vi "SwissSPAD Live_Get Next Series Step.vi"(8 "error in (no error)":errorcluster, 11 "SwissSPAD Live Internal Variables in":T1={"okCFrontPanelDevices Refnum"=refnum, "Bottom Device Refnum"=refnum, "Display Image"=refnum, "# Live Images"=0, "relative s"=0.0, "# Image Sets"=0, "Message"="", "Current Image Set"=0, "# Datasets in Series"=0, "Current Dataset"=0, "Live Mode"=FALSE, "Recording Mode"=FALSE, "Record Button"=refnum, "\nLive Button"=refnum, "SwissSPAD Live Gate Image Data Q Name"="SS2 Live Gate Data Q", "Discard First Image"=FALSE, "Image Information"={"Save ROI Only"=FALSE, "Left"=0, "Top"=0, "Right"=0, "Bottom"=0, "Use Current ROI"=FALSE}, "Image Binning Options"={"Use Image Binning"=FALSE, "X Bin"=1, "Y Bin"=1}, "Bottom FPGA Serial Number"="", "Detector PCB Version"=enum."SS2 PCB1", "# Acquisitions"=1, "10 bits"=FALSE, "Top FPGA Serial Number"="", "Top Device Refnum"=refnum} {"# Acquisitions" min=1; "Image Binning Options"."Y Bin" min=1; "Image Binning Options"."X Bin" min=1}) -> (0 "Error Out":errorcluster, 1 "Message out":string, 2 "SwissSPAD Live Atomic Action":T6[](array[typedef]), 3 "SwissSPAD Live Internal Variables out":T1={"okCFrontPanelDevices Refnum"=refnum, "Bottom Device Refnum"=refnum, "Display Image"=refnum, "# Live Images"=0, "relative s"=0.0, "# Image Sets"=0, "Message"="", "Current Image Set"=0, "# Datasets in Series"=0, "Current Dataset"=0, "Live Mode"=FALSE, "Recording Mode"=FALSE, "Record Button"=refnum, "\nLive Button"=refnum, "SwissSPAD Live Gate Image Data Q Name"="SS2 Live Gate Data Q", "Discard First Image"=FALSE, "Image Information"={"Save ROI Only"=FALSE, "Left"=0, "Top"=0, "Right"=0, "Bottom"=0, "Use Current ROI"=FALSE}, "Image Binning Options"={"Use Image Binning"=FALSE, "X Bin"=1, "Y Bin"=1}, "Bottom FPGA Serial Number"="", "Detector PCB Version"=enum."SS2 PCB1", "# Acquisitions"=1, "10 bits"=FALSE, "Top FPGA Serial Number"="", "Top Device Refnum"=refnum} {"# Acquisitions" min=1; "Image Binning Options"."Y Bin" min=1; "Image Binning Options"."X Bin" min=1})   [LabVIEW 2021]
uses:
  SwissSPAD Live_Q [Element].ctl
  SwissSPAD Live_Q Event List.ctl
  SwissSPAD Live_Internal Variables.ctl
  D:/UCLA Thinkpad Google Drive/LabVIEW 2021 SP1/builds/SwissSPAD Live Distribution/Opal Kelly/C# Wrapper/v5.0.2/libFrontPanel-csharp.dll
  Opal Kelly/C# Wrapper/v5.0.2/libFrontPanel-csharp.dll
  <vilib>/vision/Image Controls.llb/IMAQ Image.ctl
  SwissSPAD Live_Image ROI Information.ctl
  Phasor/Image Binning Options.ctl
  SwissSPAD Live_SSx PCB Version.ctl
  SwissSPAD Live_Settings List.ctl
  SwissSPAD Live_File Information.ctl
  Variant/Variant to Data/Variant to Data.lvlib
  Notebook/Notebook.lvlib
  Rich Text Box/Rich Text Box.lvlib
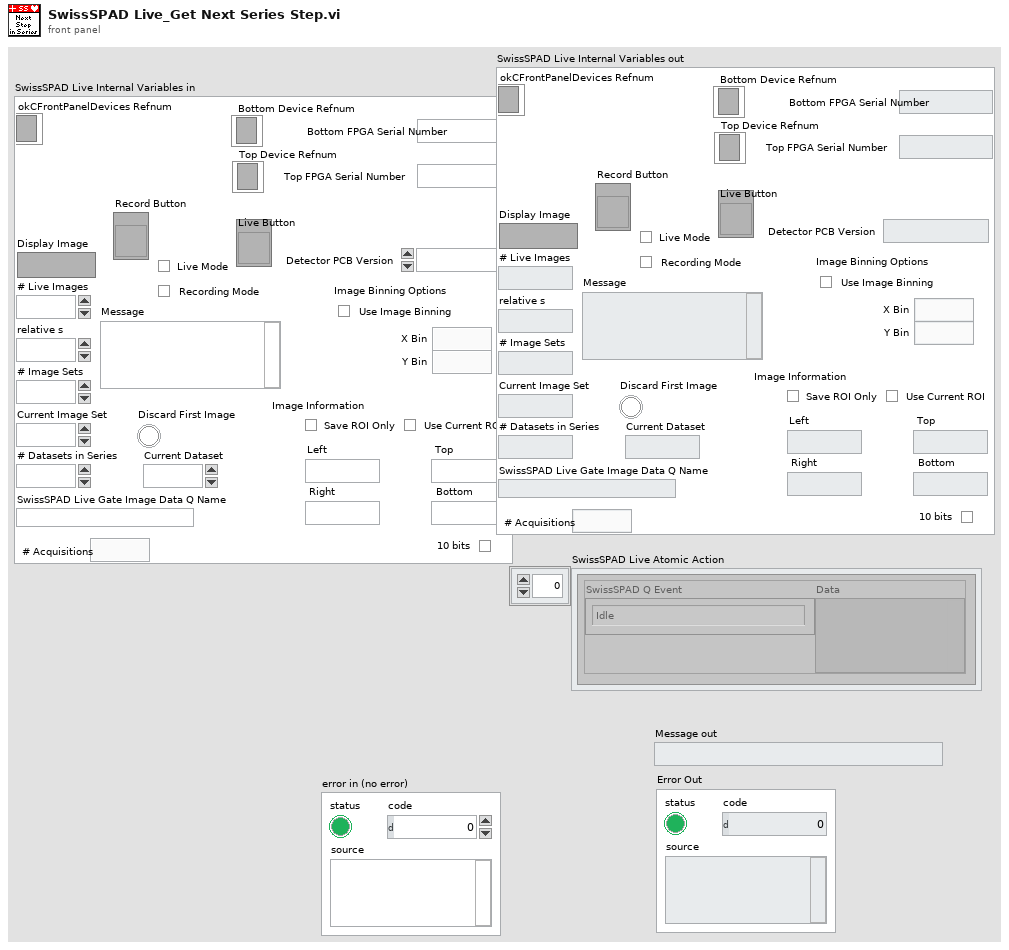
[diagram p1: front panel]
types:
  T1 = typedef "SwissSPAD Live_Internal Variables.ctl" = cluster{"okCFrontPanelDevices Refnum":refnum<k24>, "Bottom Device Refnum":refnum<k24>, "Display Image":T2, "# Live Images":i32, "relative s":dbl, "# Image Sets":i32, "Message":string, "Current Image Set":i32, "# Datasets in Series":i32, "Current Dataset":i32, "Live Mode":bool, "Recording Mode":bool, "Record Button":refnum<vi>, "\nLive Button":refnum<vi>, "SwissSPAD Live Gate Image Data Q Name":string, "Discard First Image":bool, "Image Information":T3, "Image Binning Options":T4, "Bottom FPGA Serial Number":string, "Detector PCB Version":T5, "# Acquisitions":u32, "10 bits":bool, "Top FPGA Serial Number":string, "Top Device Refnum":refnum<k24>}
  T2 = typedef "IMAQ Image.ctl" = refnum<image>
  T3 = typedef "SwissSPAD Live_Image ROI Information.ctl" = cluster{"Save ROI Only":bool, "Left":u16, "Top":u16, "Right":u16, "Bottom":u16, "Use Current ROI":bool}
  T4 = typedef "Image Binning Options.ctl" = cluster{"Use Image Binning":bool, "X Bin":i32, "Y Bin":i32}
  T5 = typedef "SwissSPAD Live_SSx PCB Version.ctl" = enum16{"unknown", "SS2 PCB1", "SS2 PCB2", "SS3 PCB1"}
  T6 = typedef "SwissSPAD Live_Q [Element].ctl" = cluster{"SwissSPAD Q Event":T7, "Data":variant}
  T7 = typedef "SwissSPAD Live_Q Event List.ctl" = enum16{"---- UI ----", "Idle", "Initialization", "Init FPGA(s)", "Init Top FPGA (deprecated)", "FPGA(s) Status", "Top FPGA Status (deprecated)", "Reset FPGA(s)", "Reset Top FPGA (deprecated)", "Refresh Display Image", "Quit", "---- DAQ ----", "Start Recording", "Start Live Acquisition", "Initialize Recording Mode", "Initialize FPGA (Live Mode)", "Get Image Set", "Get Single Image", "Update Image Display", "Stop Live Acquisition", "Stop Data Recording", "Stop Data Saving", "---- Image ----", "Copy Data to Clipboard", "Set Image Palette", "Save Displayed Image with Overlay", "Save Image Data as TIFF"}
  T8 = typedef "SwissSPAD Live_Settings List.ctl" = enum16{"FPGA:Bottom Half", "FPGA:Top Half", "FPGA:Bottom Bitfile Path", "FPGA:Top Bitfile Path", "FPGA:Bottom Bitstream Version", "FPGA:Top Bitstream Version", "FPGA:Auto Reset FPGA", "FPGA:Bottom FPGA Serial Number", "FPGA:Top FPGA Serial Number", "FPGA:Detector PCB Version", "Acquisition Parameters:Microlens", "Acquisition Parameters:SS2 DAQ Parameters", "Acquisition Parameters:Gate Configuration Array", "Acquisition Parameters:SS3 DAQ Parameters", "Acquisition Parameters:Buffer Size (# 8-bit Gates)", "File Information:File Information", "File Information:# Datasets in Series", "File Information:Scrambled File Flag", "File Information:SS3 Gate Slip Correction", "File Information:SS3 Hot Pixel Mismatch Detection", "File Information:Delay between Datasets", "File Information:Save Sum of All Gates Preview", "Image Parameters:Image ROI Information", "Image Parameters:Image Binning Options", "Image Parameters:SS3 Displayed Image", "Image Parameters:Image Display Options", "Image Parameters:Use Histogram Cursors", "Image Parameter:FPGA Data to Display", "UI Settings:Histogram Bins Number", "UI Settings:Use Image Display Options", "UI Settings:Verbose Settings", "UI Settings:Verbose Saving"}
  T9 = typedef "SwissSPAD Live_File Information.ctl" = cluster{"File Folder":path, "File Name":string, "File Index":u32, "Author":string, "Sample":string, "Compression":bool, "Compression Level":u8}
  T10 = typedef "Rich Text Box.lvlib/Text Formatting.ctl" = cluster{"Font":string, "Text Color":T11, "Text Background Color":T11, "Text Style":enum16{"Regular", "Bold", "Italic", "Underline", "Strikeout"}, "Font Size (Points)":dbl, "Text Alignment":i32}
  T11 = typedef "Rich Text Box.lvlib/Text Colors.ctl" = enum16{"Unchanged", "Black", "Blue", "Brown", "Gray", "Green", "Orange", "Pink", "Red", "White"}
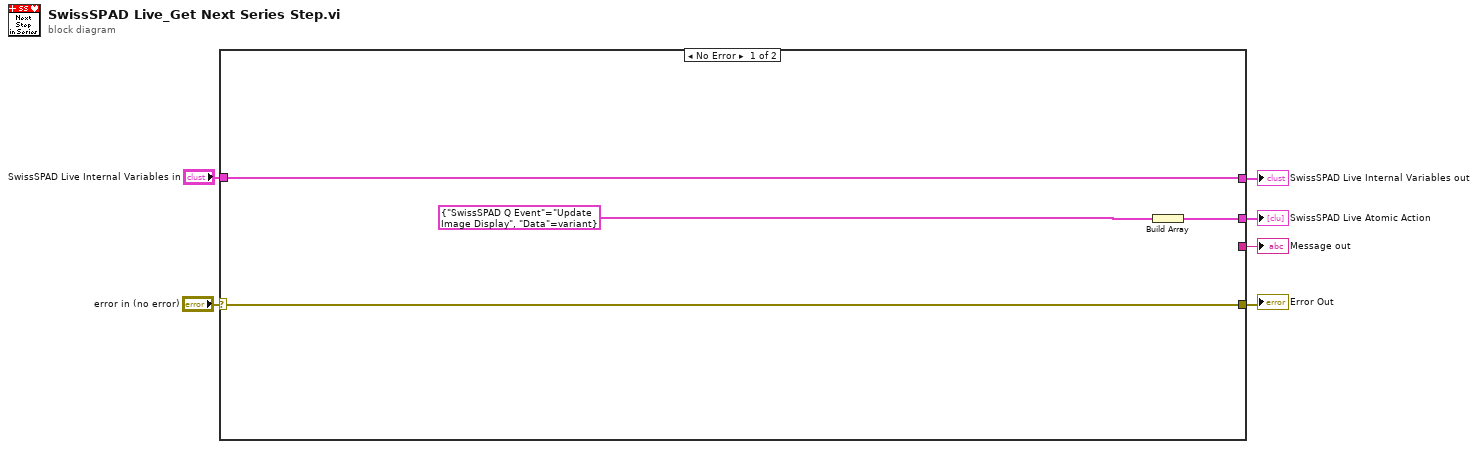
[diagram p0: block diagram]
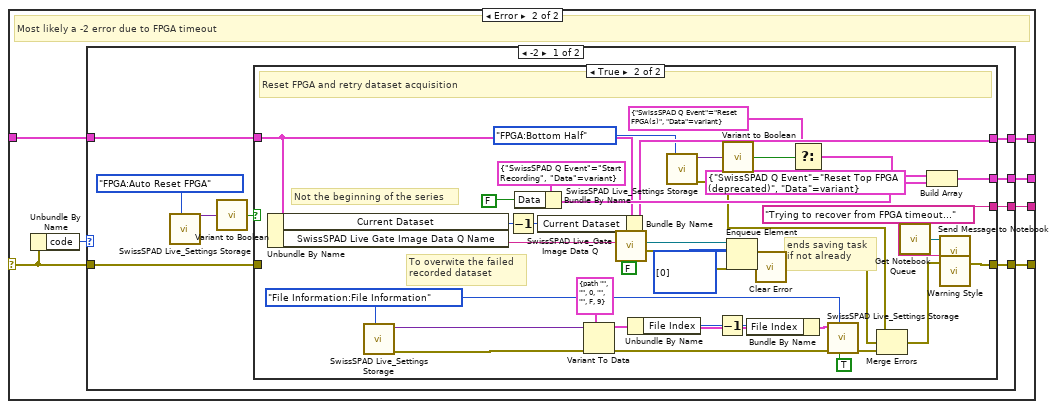
[diagram p2: hidden frame]
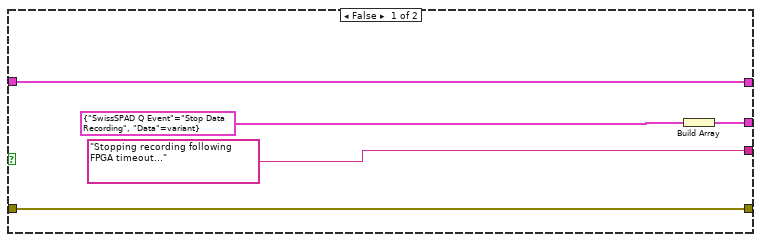
[diagram p3: hidden frame]
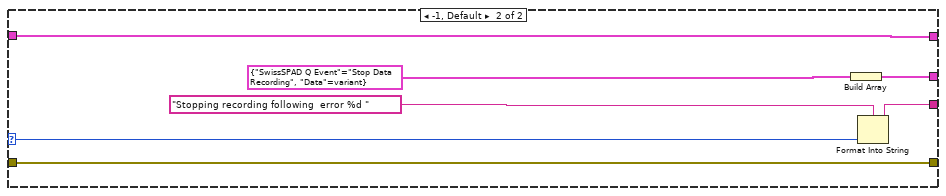
[diagram p4: hidden frame]
diagram:
  n1 = case shown="No Error" "error in (no error)" {
    selector: "error in (no error)" -> [w9 w11]
    tunnel: [w7 w17] -> w5
    tunnel: [_ w16] -> w4
    tunnel: [w9 w15] -> w3
    tunnel: "SwissSPAD Live Internal Variables in" -> [w8 w14]
    tunnel: [w8 w13] -> w1
    frame No Error {
      n2 = Build Array(T6 {"SwissSPAD Q Event"=enum."Update Image Display", "Data"=variant} ("SS2 Live Atomic Action")) -> (w7:T6[])
    }
    frame Error {
      # "Most likely a -2 error due to FPGA timeout"
      n3 = Unbundle By Name(w11) -> ("code"=w12:i32)
      n4 = case shown="-2" w12 {
        selector: w12 -> [_ w70]
        tunnel: [w26 w76] -> w17
        tunnel: [w24 w72] -> w16
        tunnel: [w23 w73] -> w15
        tunnel: w14 -> [w22 w75]
        tunnel: [w21 w75] -> w13
        tunnel: w11 -> [w20 w73]
        frame -2 {
          n5 = call "SwissSPAD Live_Settings Storage.vi"("Settings List"=SwissSPAD_Live_Settings_List."FPGA:Auto Reset FPGA") -> ("Variant Data out"=w18:variant)  [unwired: 9 in, 1 out]
          n6 = call "Variant to Boolean.vi"("Variant"=w18) -> ("Value"=w25:bool)  [unwired: 8 in]
          n7 = case shown="True" w25 {
            tunnel: [w28 w69] -> w26
            tunnel: ["Stopping recording following FPGA timeout..." ("Message out") w59] -> w24
            tunnel: [w27 w68] -> w23
            tunnel: w22 -> [w29 w48]
            tunnel: [w29 w47] -> w21
            tunnel: w20 -> [w27 _]
            frame False {
              n8 = Build Array(T6 {"SwissSPAD Q Event"=enum."Stop Data Recording", "Data"=variant} ("SS2 Live Atomic Action")) -> (w28:T6[])
            }
            frame True {
              w32 = SwissSPAD_Live_Settings_List."File Information:File Information" ("Settings List")
              w59 = "Trying to recover from FPGA timeout..." ("Message")
              # "To overwite the failed recorded dataset"
              # "ends saving task if not already"
              # "To overwite the failed recorded dataset"
              # "Not the beginning of the series"
              # "Reset FPGA and retry dataset acquisition"
              n9 = Unbundle By Name(w48) -> ("Current Dataset"=w46:i32, "SwissSPAD Live Gate Image Data Q Name"=w63:string)
              n10 = call "SwissSPAD Live_Settings Storage.vi"("Settings List"=w32) -> ("Error Out"=w57:errorcluster, "Variant Data out"=w33:variant)  [unwired: 9 in]
              n11 = Decrement(x=w46) -> (x-1=w45:i32)
              n12 = Bundle By Name(cluster=T6 {"SwissSPAD Q Event"=enum."Start Recording", "Data"=variant} ("SS2 Live Atomic Action"), "Data"=FALSE) -> (w60:T6)
              n13 = Bundle By Name(cluster=w48, "Current Dataset"=w45) -> (w47:T1)
              n14 = Variant To Data(error in=w57, type=T9 {"File Folder"=path "", "File Name"="", "File Index"=0, "Author"="", "Sample"="", "Compression"=FALSE, "Compression Level"=9} ("File Information"), Variant=w33) -> (data=w55:T9, error out=w56:errorcluster)
              n15 = call "SwissSPAD Live_Gate Image Data Q.vi"("create if not found? (T)"=FALSE, "SwissSPAD Live Gate Image Data Q Name"=w63) -> ("error out"=w38:errorcluster, "SwissSPAD Live Gate Image Data Q"=w65:refnum<queue>)  [unwired: 7 in, 1 out]
              n16 = Unbundle By Name(w55) -> ("File Index"=w54:u32)
              n17 = call "SwissSPAD Live_Settings Storage.vi"("Settings List"=SwissSPAD_Live_Settings_List."FPGA:Bottom Half") -> ("Error Out"=w43:errorcluster, "Variant Data out"=w34:variant)  [unwired: 9 in]
              n18 = Decrement(x=w54) -> (x-1=w53:u32)
              n19 = call "Variant to Boolean.vi"("Variant"=w34) -> ("Value"=w42:bool)  [unwired: 8 in]
              n20 = Enqueue Element(queue=w65, element=u8[][] [[0]], error in (no error)=w38) -> (error out=w49:errorcluster)  [unwired: 1 in, 2 out]
              n21 = Bundle By Name(cluster=w55, "File Index"=w53) -> (w36:T9)
              n22 = call "Clear Error.vi"("Error In"=w49) -> ("no Error Out"=w37:errorcluster)  [unwired: 8 in]
              n23 = Select(t=T6 {"SwissSPAD Q Event"=enum."Reset FPGA(s)", "Data"=variant} ("element"), s=w42, f=T6 {"SwissSPAD Q Event"=enum."Reset Top FPGA (deprecated)", "Data"=variant} ("element")) -> (s? t:f=w39:T6)
              n24 = call "SwissSPAD Live_Settings Storage.vi"("Set/Get(F)"=TRUE, "Settings List"=w32, "Error In"=w56, "Variant Data in"=w36) -> ("Error Out"=w51:errorcluster)  [unwired: 6 in, 1 out]
              n25 = Merge Errors(w43, w37, w51) -> (w50:errorcluster)
              n26 = call "Get Notebook Queue.vi"() -> ("Notebook Queue"=w67:refnum<queue>)  [unwired: 9 in]
              n27 = Build Array(w39, w60) -> (w69:T6[])
              n28 = call "Warning Style.vi"() -> ("Error Formatting"=w66:T10)
              n29 = call "Send Message to Notebook.vi"("Text Formatting"=w66, "Error In"=w50, "Message"=w59, "Notebook Queue"=w67) -> ("Error Out"=w68:errorcluster)  [unwired: 4 in, 1 out]
            }
          }
        }
        frame -1, Default {
          n30 = Build Array(T6 {"SwissSPAD Q Event"=enum."Stop Data Recording", "Data"=variant} ("SS2 Live Atomic Action")) -> (w76:T6[])
          n31 = Format Into String(format string="Stopping recording following  error %d " ("Message out"), w70) -> (resulting string=w72:string)  [unwired: 2 in, 1 out]
        }
      }
    }
  }
  "SwissSPAD Live Atomic Action" <- w5
  "Error Out" <- w3
  "Message out" <- w4
  "SwissSPAD Live Internal Variables out" <- w1
